vi "Extrinsic_inverse.vi"(7 "resolution":i32[](array[numeric]), 10 "extrinsic":dbl[][](array[numeric]), 11 "X'":dbl[][](array[numeric])) -> (3 "X'":dbl[][](array[numeric]))   [LabVIEW 2017]
uses:
  <vilib>/Analysis/Matrix/Numeric/Conversions/Matrix To Array - RM.vi
  <vilib>/Analysis/Matrix/Numeric/Conversions/Array To Matrix - RA2.vi
  <vilib>/Analysis/baseanly.llb/Real Inverse Matrix.vi
  <vilib>/Analysis/Matrix/Numeric/Multiply/Multiply - RM,RM.vi
  <vilib>/Analysis/NI_AALBase.lvlib
  <vilib>/Analysis/Matrix/NI_Matrix.lvlib
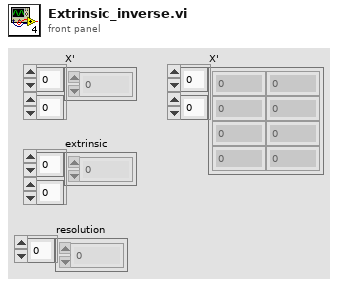
[diagram p1: front panel]
types:
  T1 = typedef "NI_Matrix.lvlib/RealMatrix.ctl" = dbl[][]
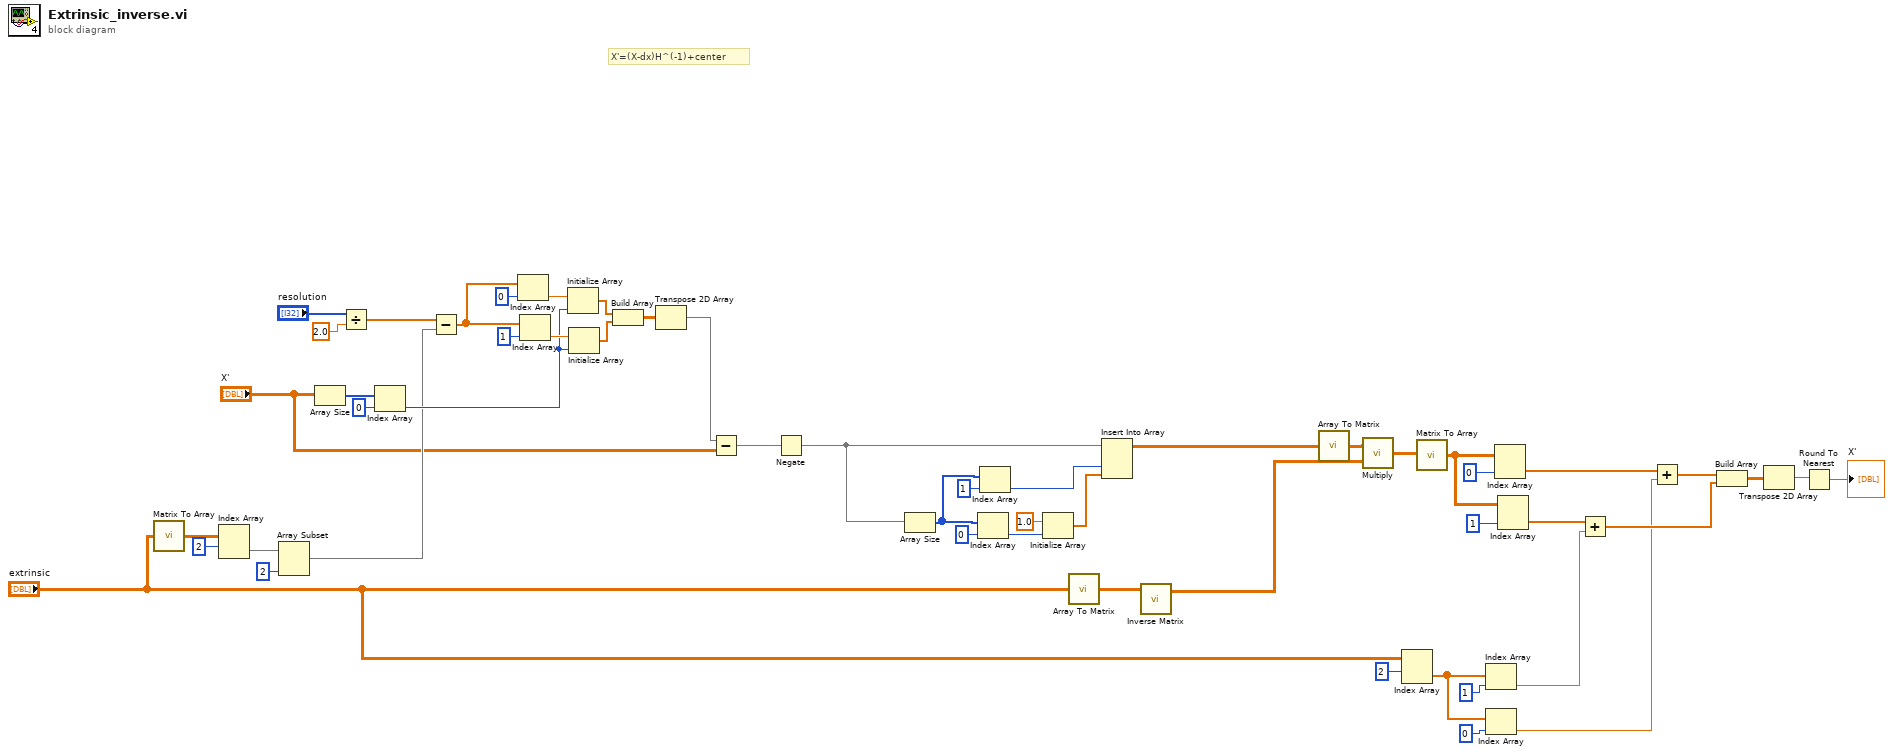
[diagram p0: block diagram]
diagram:
  # "X'=(X-dx)H^(-1)+center"
  n1 = call-poly <vilib>:"Matrix To Array.vi"("Real Matrix"="extrinsic") -> ("Real 2D Array"=w7:dbl[][])
  n2 = Index Array(array=w7, index (row)=2) -> (element=w8:dbl[])  [unwired: 1 in]
  n3 = Array Subset(array=w8, length=2) -> (w6:dbl[])  [unwired: 1 in]
  n4 = Array Size(array="X'") -> (size(s)=w12:i32[])
  n5 = Divide(x="resolution", y=2.0) -> (x/y=w23:dbl[])
  n6 = Index Array(array=w12, index=0) -> (element=w11:i32)
  n7 = Subtract(x=w23, y=w6) -> (x-y=w22:dbl[])
  n8 = Index Array(array=w22, index=0) -> (element=w19:dbl)
  n9 = Index Array(array=w22, index=1) -> (element=w18:dbl)
  n10 = Initialize Array(w19, w11) -> (w17:dbl[])
  n11 = Initialize Array(w18, w11) -> (w16:dbl[])
  n12 = Build Array(w17, w16) -> (w15:dbl[][])
  n13 = Transpose 2D Array(2D array=w15) -> (transposed array=w4:dbl[][])
  n14 = Subtract(x=w4, y="X'") -> (x-y=w2:dbl[][])
  n15 = Negate(x=w2) -> (-x=w1:dbl[][])
  n16 = Array Size(array=w1) -> (size(s)=w48:i32[])
  n17 = Index Array(array=w48, index=0) -> (element=w47:i32)
  n18 = Index Array(array=w48, index=1) -> (element=w50:i32)
  n19 = Initialize Array(1.0 ("element"), w47) -> (w46:dbl[])
  n20 = call-poly <vilib>:"Array To Matrix.vi"("Real 2D Array"="extrinsic") -> ("Real Matrix"=w26:T1)
  n21 = Insert Into Array(array=w1, index (col)=w50, new element=w46) -> (w45:dbl[][])  [unwired: 1 in]
  n22 = call-poly <vilib>:"Inverse Matrix.vi"("Input Matrix"=w26) -> ("Inverse Matrix"=w25:T1)  [unwired: 1 in, 1 out]
  n23 = call-poly <vilib>:"Array To Matrix.vi"("Real 2D Array"=w45) -> ("Real Matrix"=w44:T1)
  n24 = call-poly <vilib>:"Multiply.vi"("Real Matrix B"=w25, "Real Matrix A"=w44) -> ("A * B"=w27:T1)
  n25 = Index Array(array="extrinsic", index (row)=2) -> (element=w31:dbl[])  [unwired: 1 in]
  n26 = call-poly <vilib>:"Matrix To Array.vi"("Real Matrix"=w27) -> ("Real 2D Array"=w34:dbl[][])
  n27 = Index Array(array=w31, index=1 ("index (row)")) -> (element=w36:dbl)
  n28 = Index Array(array=w31, index=0 ("index (row)")) -> (element=w38:dbl)
  n29 = Index Array(array=w34, index (col)=0 ("index (row)")) -> (element=w37:dbl[])  [unwired: 1 in]
  n30 = Index Array(array=w34, index (col)=1 ("index (row)")) -> (element=w35:dbl[])  [unwired: 1 in]
  n31 = Add(x=w35, y=w36) -> (x+y=w40:dbl[])
  n32 = Add(x=w37, y=w38) -> (x+y=w39:dbl[])
  n33 = Build Array(w39, w40) -> (w41:dbl[][])
  n34 = Transpose 2D Array(2D array=w41) -> (transposed array=w51:dbl[][])
  n35 = Round To Nearest(number=w51) -> (nearest integer value=→"X'":dbl[][])
